vi "Initialize.vi"(7 "I2C Channel":u8, 8 "error in (no error)":errorcluster, 11 "LINX Resource In":T1) -> (0 "error out":errorcluster, 3 "LINX Resource Out":T1)   [LabVIEW 2014, in "LMH-LINX.lvlib" / "HMC6352.lvlib"]
uses:
  <vilib>/MakerHub/LINX/Public/Sensors/Orientation/Compass/HMC6352/HMC6352.lvlib
  <vilib>/MakerHub/LINX/Private/Type Defs/LINX Ref.ctl
  <vilib>/MakerHub/LINX/Private/Type Defs/Platform.ctl
  <vilib>/MakerHub/LINX/Private/Type Defs/Interface.ctl
  <vilib>/MakerHub/LINX/Private/Device/Type Defs/LINX Device Config.ctl
  <vilib>/MakerHub/LINX/Private/Device/Type Defs/TCP Config.ctl
  <vilib>/MakerHub/LINX/Private/Device/Type Defs/Channels.ctl
  <vilib>/MakerHub/LINX/LMH-LINX.lvlib
  <vilib>/MakerHub/LINX/Private/Device/Device.lvlib
panel:
  # "INPUTS"
  # "OUTPUTS"
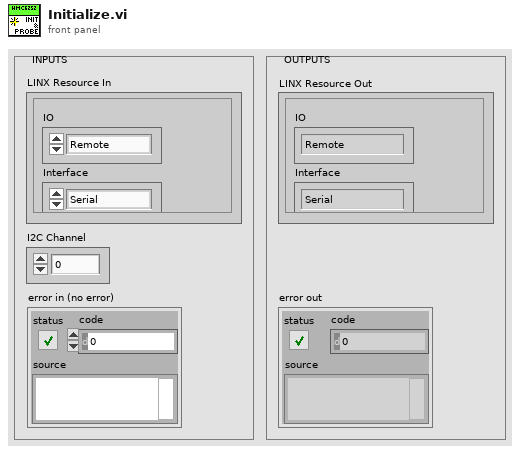
[diagram p1: front panel]
types:
  T1 = typedef "LMH-LINX.lvlib/LINX Ref.ctl" = cluster{"IO":T2, "Interface":T3, "LINX Device Config":T4}
  T2 = typedef "LMH-LINX.lvlib/Platform.ctl" = enum16{"Remote", "Local"}
  T3 = typedef "LMH-LINX.lvlib/Interface.ctl" = enum16{"Serial", "TCP"}
  T4 = typedef "LMH-LINX.lvlib/Device.lvlib/LINX Device Config.ctl" = cluster{"Interface":T3, "COM Port":refnum<visa-resource-name>, "TCP Configuration":T5, "Device Family":u8, "Device ID":u8, "Device Name":string, "TCP Ref":refnum<k5>, "Channels":T6}
  T5 = typedef "LMH-LINX.lvlib/Device.lvlib/TCP Config.ctl" = cluster{"IP Address":string, "Port":u16}
  T6 = typedef "LMH-LINX.lvlib/Channels.ctl" = cluster{"DI":u8[], "DO":u8[], "AI":u8[], "AO":u8[], "PWM":u8[], "QE":u8[], "UART":u8[], "I2C 2":u8[], "SPI":u8[], "CAN":u8[], "Servo":u8[], "AI Ref (V)":dbl, "AI Resolution (Bits)":u8, "AO Ref (V)":dbl, "AO Resolution (Bits)":u8}
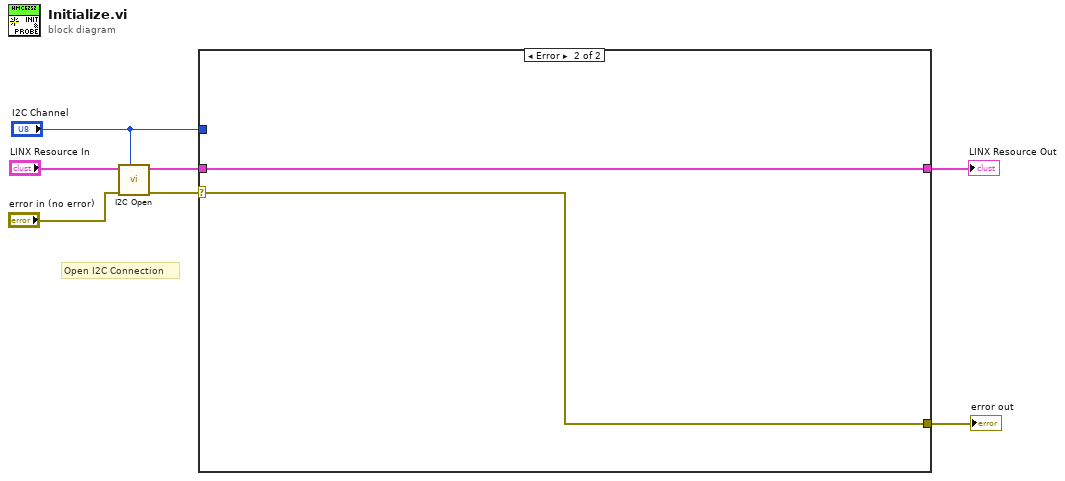
[diagram p0: block diagram]
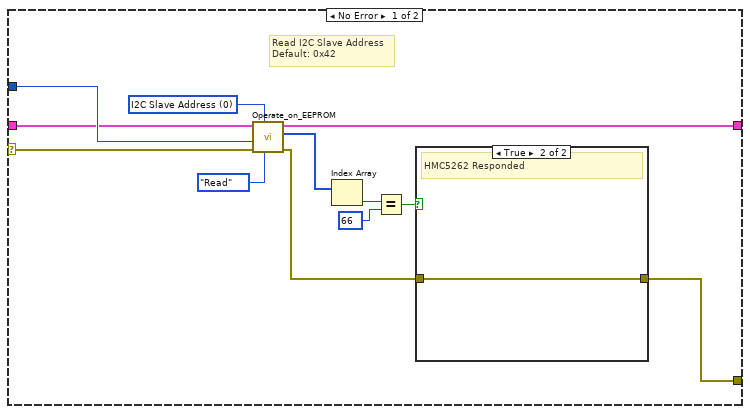
[diagram p2: hidden frame]
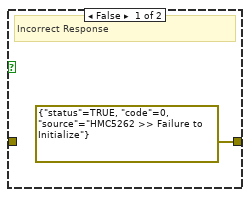
[diagram p3: hidden frame]
diagram:
  # "Open I2C Connection"
  n1 = call <vilib>:"I2C Open.vi"("I2C Channel (0)"="I2C Channel", "Error In"="error in (no error)", "LINX Resource"="LINX Resource In") -> ("Error Out"=w2:errorcluster, "LINX Resource"=w4:T1)  [unwired: 7 in]
  n2 = case shown="Error" w2 {
    selector: w2 -> [w9 w23]
    tunnel: [w11 w23] -> w7
    tunnel: w4 -> [w8 w22]
    tunnel: [w10 w22] -> w6
    tunnel: "I2C Channel" -> [w19 _]
    frame No Error {
      w17 = u8 0 items=["I2C Slave Address", "Magnetometer X Offset MSB", "Magnetometer X Offset LSB", "Magnetometer Y Offset MSB", "Magnetometer Y Offset LSB", "Measurement Time Delay", "Number of Summed Measurements", "Software Version Number", "Operation Mode Byte"] ("EEPROM Addresses")
      # "Read I2C Slave Address\nDefault: 0x42"
      n3 = call <vilib>:"Operate_on_EEPROM.vi"("Operation"=enum16{"Write", "Read"}."Read", "EEPROM Addresses"=w17, "error in (no error)"=w9, "I2C Channel"=w19, "LINX Resource In"=w8) -> ("error out"=w12:errorcluster, "Data Out"=w16:u8[], "LINX Resource Out"=w10:T1)  [unwired: 4 in]
      n4 = Index Array(array=w16) -> (element=w15:u8)  [unwired: 1 in]
      n5 = Equal?(x=w15, y=u8 66) -> (x = y?=w13:bool)
      n6 = case shown="True" w13 {
        tunnel: w12 -> [_ w21]
        tunnel: [errorcluster {"status"=TRUE, "code"=0, "source"="HMC5262 >> Failure to Initialize"} ("error out") w21] -> w11
        frame False {
          # "Incorrect Response"
        }
        frame True {
          # "HMC5262 Responded"
        }
      }
    }
    frame Error {
    }
  }
  "error out" <- w7
  "LINX Resource Out" <- w6
